vi "数组排序.vi"() -> ()   [LabVIEW 2018]
uses:
  9a49b940-4c72-48fa-9163-e8ab85f8d955.vi
  <vilib>/Array/Sort 2D Array - Pop Stack.vi
  <vilib>/Array/Sort 2D Array - Push Stack.vi
panel:
  out "字符串":string
  in  "index":i32 caption="索引"
  in  "dimension to index (column)":enum16{"column", "row"}(ring) caption="要索引的维度（列）"
  out "排序后二维数组":dbl[][](array[numeric])
  in  "二维数组":dbl[][](array[numeric])
  in  "停止":bool
  out "排序后数组":dbl[](array[numeric])
  in  "数组":dbl[](array[numeric])
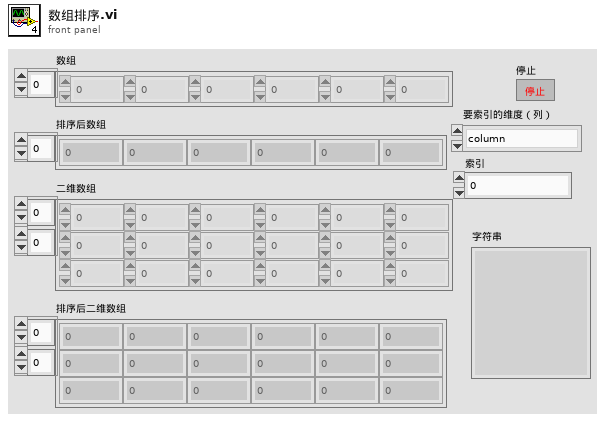
[diagram p1: front panel]
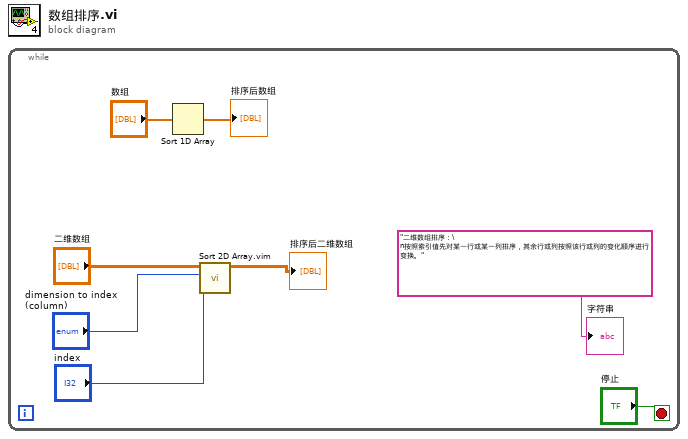
[diagram p0: block diagram]
diagram:
  n1 = while {
    stop <- "停止" stop-if-true
    n2 = Sort 1D Array(array="数组") -> (sorted array=→"排序后数组":dbl[])
    n3 = call "Sort 2D Array.vim"("index"="index", "dimension to index (column)"="dimension to index (column)", "2D array"="二维数组") -> ("sorted 2D array"=→"排序后二维数组":dbl[][])  [unwired: 7 in, 1 out]
    "字符串" <- "二维数组排序：\n按照索引值先对某一行或某一列排序，其余行或列按照该行或列的变化顺序进行变换。"
  }
